vi "Intake IR.vi"(7 "Unload?":bool, 11 "Speed":dbl) -> (3 "Speeeeeeed":dbl, 5 "Rollers Enabled?":bool)   [LabVIEW 2015]
uses:
  Common Code/Intake Commands Cluster.ctl
  Common Code/Intake Commands.ctl
  Common Code/Intake Mode.ctl
  Common Code/Change Detect Boolean.vi
  Robot Global Data.vi
panel:
  in  "Intake Commands Cluster":T1={"Intake Commands"=enum."Load", "Intake Mode"=enum."Auto", "Override IR"=FALSE, "Angle Target"=0.0}
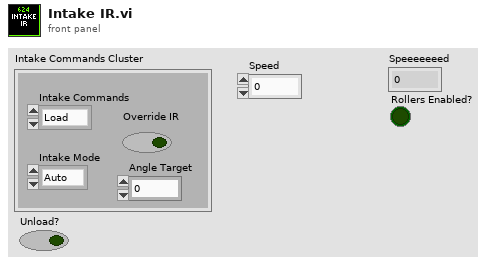
[diagram p1: front panel]
types:
  T1 = typedef "Intake Commands Cluster.ctl" = cluster{"Intake Commands":T2, "Intake Mode":T3, "Override IR":bool, "Angle Target":dbl}
  T2 = typedef "Intake Commands.ctl" = enum16{"Settle Ball", "Unload", "Load", "Pull up", "Drop low", "Idle", "Lift Half", "Go To Angle"}
  T3 = typedef "Intake Mode.ctl" = enum16{"Safe", "Auto", "Manual"}
  T4 = typedef "Dashboard Control Data.ctl" = cluster{"Shooter Presets":T5, "Encoder Control":T7, "Steer PID output":cluster{"output high":dbl, "output low":dbl}, " Steer PID gains":cluster{"proportional gain (Kc)":dbl, "integral time (Ti, min)":dbl, "derivative time (Td, min)":dbl}, "Drivetrain Settings":T8, "Vision Packet":T9, "Dashboard Drivetrain Command":T10, "Info/Command Cluster":T12, "Ball Vision Packet":T13, "Intake Presets":T15, "Intake Encoder Control":T17, "Climb Presets":T18, "Goal Output Range":cluster{"output high":dbl, "output low":dbl}, "Enabled Systems":T19, "Auton Presets":T20, "Pressure M":dbl, "Pressure B":dbl, "Vision Timeout":dbl, "Auto-Shift":T21, "Catapult Setpoints":T22}
  T5 = typedef "Shooter Presets.ctl" = cluster{"Batter Shot":T6, "Deep Middle":T6, "Manual Shot":T6, "Left Ticks Per Rotation":dbl, "Right Ticks Per Rotation":dbl, "Low Bar Shot":T6, "Shooter RPM Tolerance":dbl, "Trigger Power":dbl, "Fire from Load Delay":i32, "Max Angle":dbl, "Min Angle":dbl, "Angle PID gains":cluster{"P":dbl, "I":dbl, "D":dbl}, "Angle Output":cluster{"output high":dbl, "output low":dbl}, "Shooter Angle Tolerance":dbl, "Vision Shoot x^2":dbl, "Vision Shoot x":dbl, "Feed Forward Max Accel":dbl, "Feed Forward Kv":dbl, "Backwards Trigger":dbl, "Shot Finish Delay (ms)":dbl, "Angle Max Current":dbl, "Angle Current Trip Time":dbl, "Intake Angle":dbl, "Vision Shoot c":dbl, "Reset?":bool, "Button Release Delay":dbl, "Angle Pot x":dbl, "Angle Pot c":dbl, "Ignore Angle?":bool, "Max RPM":dbl, "Safty Frist Angle":dbl, "Intake Danger Height":dbl, "Angle Pot B":i32, "Angle Pot M":dbl, "FF Finish RPM":dbl, "RPM PID Right":cluster{"P":dbl, "I":dbl, "D":dbl, "FF":dbl}, "RPM PID Left":cluster{"P":dbl, "I":dbl, "D":dbl, "FF":dbl}, "Backwards RPM":dbl, "Vision RPM":dbl, "Run Wheels Backward Delay":u32, "Cleat Shot":T6, "Vision Far RPM":dbl, "Vision Far Distance":dbl, "Vision Far Angle":dbl}
  T6 = typedef "Shot Presets.ctl" = cluster{"L":dbl, "R":dbl, "A":dbl}
  T7 = typedef "Encoder Control.ctl" = cluster{"Right Tick Constant":dbl, "Left Tick Constant":dbl, "Reset?":bool, "Y Dist":cluster{"PID gains":cluster{"proportional gain (Kc)":dbl, "integral time (Ti, min)":dbl, "derivative time (Td, min)":dbl}}, "Y Stop Thresh":dbl, "Y Stop Speed":dbl}
  T8 = typedef "Drivetrain Settings.ctl" = cluster{"Gyro Tolerance":dbl, "Throttle Ramp (ms)":dbl, "Kv":dbl, "Ka":dbl, "Feed Forward P":dbl, "Feed Forward D":dbl, "Goal Vision PID gains":cluster{"proportional gain (Kc)":dbl, "integral time (Ti, min)":dbl, "derivative time (Td, min)":dbl}, "Goal Detection Window":dbl, "Creep Rate":dbl, "Vision Throttle Threshold":dbl, "Min Turn Output":dbl, "Left Batter Angle":dbl, "Right Batter Angle":dbl}
  T9 = typedef "Goal Vision Packet.ctl" = cluster{"Distance":dbl, "Center X":dbl, "Center Y":dbl, "Found Target?":bool, "Robot Center":dbl, "Angle":dbl}
  T10 = typedef "Dashboard Drivetrain Command.ctl" = cluster{"Drivetrain Vision":T11}
  T11 = typedef "Drivetrain Vision.ctl" = cluster{"Goal Window":dbl, "Ball Window":dbl}
  T12 = typedef "Ball Tracking Command Cluster.ctl" = cluster{"Distance to Ball":dbl, "Desired Angle":dbl, "Command":enum16{"Turn to Ball", "Turn to Angle", "Get Distance"}, "Pixels from Center":dbl}
  T13 = typedef "Ball Vision Packet.ctl" = cluster{"Ball Detected?":bool, "Distance to Ball":dbl, "Desired Angle":dbl, "Pixels from Center":dbl, "Tracking mode":T14}
  T14 = typedef "Tracking Mode.ctl" = enum16{"Turn to Ball", "Turn to Angle"}
  T15 = typedef "Intake Presets.ctl" = cluster{"Intake Speed":dbl, "Outake Speed":dbl, "Low Height":dbl, "Half Height":dbl, "High Idle Height":dbl, "Angle Speed":dbl, "Angle Tolerance":dbl, "Encoder Scale":dbl, "Load Height":dbl, "Output Range":T16, "Rotation Power Max/Min":dbl, "MaxCurrent":dbl, "Intake Trip Time":dbl, "Idle Height":dbl, "Max Height":dbl, "Reset Encoders?":bool, "PID gains":cluster{"proportional gain (Kc)":dbl, "integral time (Ti, min)":dbl, "derivative time (Td, min)":dbl}, "Intake Stop Delay":u32, "Settle Time":dbl, "Settle Wait Time":dbl, "Pull Up Delay":dbl}
  T16 = typedef "Drivetrain Output Range.ctl" = cluster{"output high":dbl, "output low":dbl}
  T17 = typedef "IntakeEcoderControl.ctl" = cluster{"Arm Tick Constant":dbl, "Reset?":bool, "Y Dist":cluster{"PID gains":cluster{"proportional gain (Kc)":dbl, "integral time (Ti, min)":dbl, "derivative time (Td, min)":dbl}}, "Y Stop Thresh":dbl, "Y Stop Speed":dbl}
  T18 = typedef "Climb Presets.ctl" = cluster{"Pull Power":dbl, "Extend Power":dbl}
  T19 = typedef "Enabled Systems.ctl" = cluster{"Shoot":bool, "Intake":bool, "DT":bool, "Gyro":bool, "100ms":bool, "US":bool}
  T20 = typedef "Autonomous Presets.ctl" = cluster{"Pitch Limit":dbl, "Roll Limit":dbl, "Start Position":dbl, "Cross Position":dbl}
  T21 = typedef "Auto Shift Cluster.ctl" = cluster{"Delay":dbl, "Speed Thresh":dbl, "Upshift Accel":dbl, "Upshift Throttle":dbl, "Upshift Throttle Accel":dbl, "Downshift Throttle":dbl, "Downshift Throttle Accel":dbl, "Pressure Threshold":dbl}
  T22 = typedef "Catapult Presets.ctl" = cluster{"Intake Danger Height":dbl, "Ball Security Delay ":dbl, "High PSI Minimum":dbl, "Shot Finish Delay":dbl, "Low PSI Minimum":dbl}
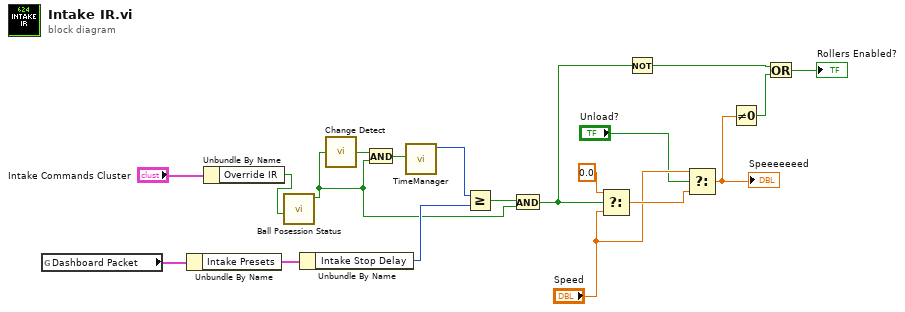
[diagram p0: block diagram]
diagram:
  n1 = global read "Robot Global Data.vi" "Dashboard Packet"() -> (w12:T4)
  n2 = Unbundle By Name(w12) -> ("Intake Presets"=w11:T15)
  n3 = Unbundle By Name("Intake Commands Cluster") -> ("Override IR"=w2:bool)
  n4 = call "Ball Posession Status.vi"("Logical Exit?"=w2) -> ("Ball Posessed?"=w1:bool)  [unwired: 10 in]
  n5 = Unbundle By Name(w11) -> ("Intake Stop Delay"=w10:u32)
  n6 = call-poly "Change Detect.vi"("In"=w1) -> ("Changed?"=w15:bool)
  n7 = And(x=w15, y=w1) -> (x .and. y?=w14:bool)
  n8 = call "TimeManager.vi"("Reset?"=w14) -> ("Time Since Reset"=w13:u32)  [unwired: 9 in, 1 out]
  n9 = Greater Or Equal?(x=w13, y=w10) -> (x >= y?=w8:bool)
  n10 = And(x=w8, y=w1) -> (x .and. y?=w4:bool)
  n11 = Select(t=0.0, s=w4, f="Speed") -> (s? t:f=w17:dbl)
  n12 = Not(x=w4) -> (.not. x?=w3:bool)
  n13 = Select(t="Speed", s="Unload?", f=w17) -> (s? t:f=w6:dbl)
  "Speeeeeeed" <- w6
  n14 = Not Equal To 0?(x=w6) -> (x != 0?=w5:bool)
  n15 = Or(x=w3, y=w5) -> (x .or. y?=→"Rollers Enabled?":bool)
